vi "读取-TCP通信功能码（参考）.vi"(8 "error in (no error)":errorcluster caption="错误输入（无错误）", 11 "设备终端输入":refnum<class "设备终端.lvclass">) -> (0 "error out":errorcluster caption="错误输出", 2 "TCP通信功能码（参考）":T1(ring), 3 "设备终端输出":refnum<class "设备终端.lvclass">)   [LabVIEW 2013, in "设备终端.lvclass"]
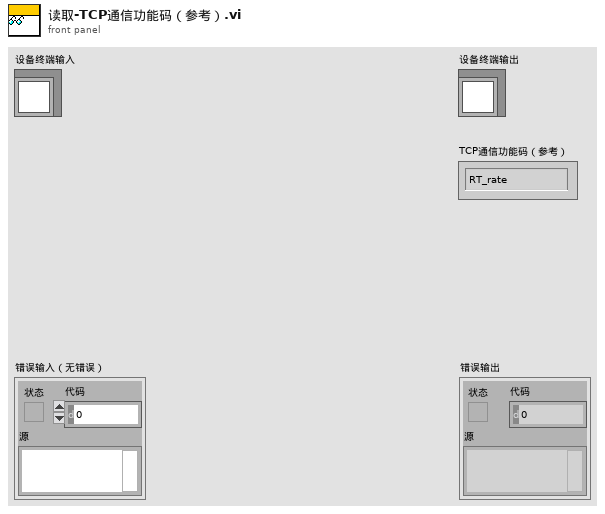
[diagram p1: front panel]
types:
  T1 = enum16{"RT_rate", "RT_dose", "set_th_rate", "set_th_dose", "set_time", "find_div_sign"}
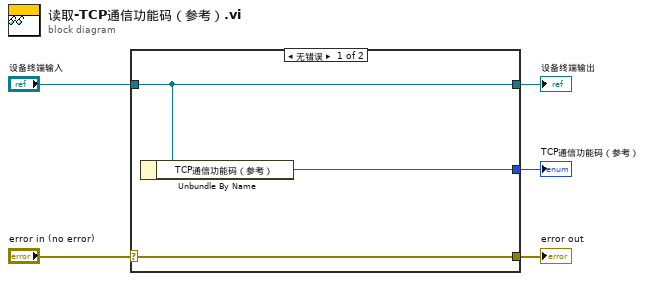
[diagram p0: block diagram]
diagram:
  n1 = case shown="无错误" "error in (no error)" {
    selector: "error in (no error)" -> [w8 w9]
    tunnel: [w8 w9] -> w4
    tunnel: [w7 w10] -> w2
    tunnel: "设备终端输入" -> [w7 w10]
    tunnel: [w6 _] -> w1
    frame No Error {
      n2 = Unbundle By Name(w7) -> ("TCP通信功能码（参考）"=w6:T1)
    }
    frame Error {
    }
  }
  "error out" <- w4
  "设备终端输出" <- w2
  "TCP通信功能码（参考）" <- w1
